vi "load_waypoint_icons.vi"() -> (3 "Waypoint Icon Reference":T1)   [LabVIEW 2013]
doc: "Loads the boat icon for use on the map. Also, replaces all the black pixels with transparent pixels.\n\n4/5/2014\nMac-I Crowell"
uses:
  TypeDef/waypoint_icon_references.ctl
  <vilib>/vision/Image Controls.llb/IMAQ Image.ctl
panel:
  out "Sailing Point Image":T2(plugin-control)
  out "Mission Image":T2(plugin-control)
  out "appended boat icon path":path
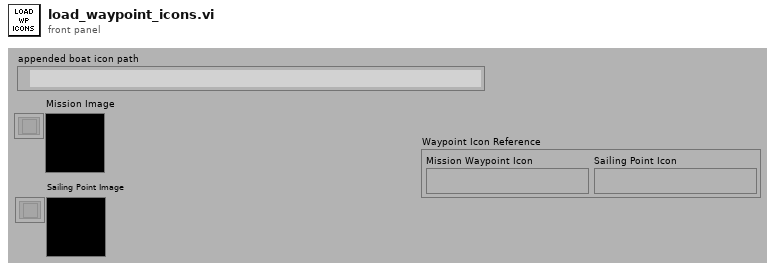
[diagram p1: front panel]
types:
  T1 = typedef "waypoint_icon_references.ctl" = cluster{"Mission Waypoint Icon":T2, "Sailing Point Icon":T2}
  T2 = typedef "IMAQ Image.ctl" = refnum<image>
  T3 = typedef "Image Type" = u32
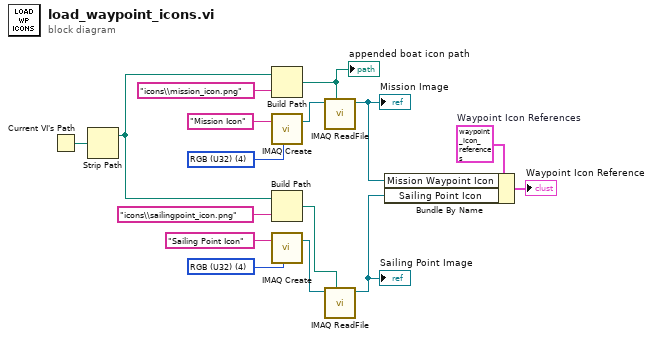
[diagram p0: block diagram]
diagram:
  w2 = T1 {"Mission Waypoint Icon"=refnum, "Sailing Point Icon"=refnum}  # Waypoint Icon References
  w6 = T3 4 items=["Grayscale (U8)", "Grayscale (I16)", "Grayscale (SGL)", "Complex (CSG)", "RGB (U32)", "HSL (U32)", "RGB (U64)", "Grayscale (U16)"] ("Image Type")
  w16 = T3 4 items=["Grayscale (U8)", "Grayscale (I16)", "Grayscale (SGL)", "Complex (CSG)", "RGB (U32)", "HSL (U32)", "RGB (U64)", "Grayscale (U16)"] ("Image Type")
  n1 = Current VI's Path() -> (path=w13:path)
  n2 = Strip Path(path=w13) -> (stripped path=w4:path)  [unwired: 1 out]
  n3 = Build Path(base path=w4, name or relative path="icons\\mission_icon.png") -> (appended path=w11:path)
  "appended boat icon path" <- w11
  n4 = call "IMAQ Create"("Image Name"="Mission Icon", "Image Type"=w16) -> ("New Image"=w14:T2)  [unwired: 2 in, 2 out]
  n5 = Build Path(base path=w4, name or relative path="icons\\sailingpoint_icon.png") -> (appended path=w10:path)
  n6 = call "IMAQ Create"("Image Name"="Sailing Point Icon", "Image Type"=w6) -> ("New Image"=w8:T2)  [unwired: 2 in, 2 out]
  n7 = call "IMAQ ReadFile"("File Path"=w11, "Image"=w14) -> ("Image Out"=w5:T2)  [unwired: 3 in, 6 out]
  "Mission Image" <- w5
  n8 = call "IMAQ ReadFile"("File Path"=w10, "Image"=w8) -> ("Image Out"=w3:T2)  [unwired: 3 in, 6 out]
  "Sailing Point Image" <- w3
  n9 = Bundle By Name(cluster=w2, "Mission Waypoint Icon"=w5, "Sailing Point Icon"=w3) -> (→"Waypoint Icon Reference":T1)
